vi "exec.vi"(8 "error in (no error)":errorcluster, 10 "context":refnum<class "Context.lvclass">, 11 "EnableMotion in":refnum<class "EnableMotion.lvclass">) -> (0 "error out":errorcluster, 2 "context 2":refnum<class "Context.lvclass">, 3 "EnableMotion out":refnum<class "EnableMotion.lvclass">)   [LabVIEW 2013, in "EnableMotion.lvclass"]
uses:
  EnableMotion.lvclass
  Context/Context.lvclass
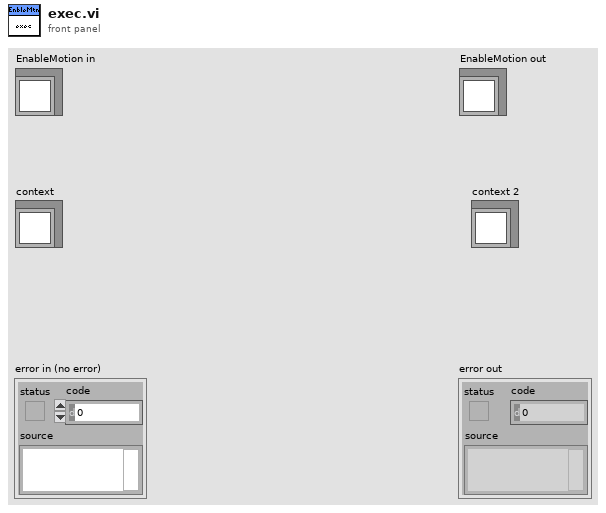
[diagram p1: front panel]
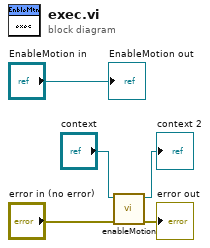
[diagram p0: block diagram]
diagram:
  n1 = call "enableMotion.vi"("error in (no error)"="error in (no error)", "Context in"="context") -> ("error out"=→"error out":errorcluster, "Context out"=→"context 2":refnum<class "Context.lvclass">)  [unwired: 8 in]
  "EnableMotion out" <- "EnableMotion in"
